vi "PID control XYZ R.vi"(0 "location":T2, 1 "x polarity":bool=TRUE, 2 "y polarity":bool, 3 "z polarity":bool, 5 "large deviation override":T1={"x (um)"=60.0, "y (um)"=80.0, "Poverride"=1.2}, 9 "deadband (um)":dbl=2.0, 11 "reinitialize? (F)":bool, 12 "XY pos range (um)":cluster{"output high":dbl, "output low":dbl}={"output high"=1000.0, "output low"=-1000.0} {"output low" format="%.2f"; "output high" format="%.2f"}, 13 "z position range (um)":cluster{"output high":dbl, "output low":dbl}={"output high"=100.0, "output low"=-100.0} {"output low" format="%.2f"; "output high" format="%.2f"}, 14 "XY gains":T3={"proportional gain (Kc)"=0.7, "integral time (Ti, sec)"=1.0, "derivative time (Td, sec)"=0.0} {"derivative time (Td, sec)" format="%.3f"; "integral time (Ti, sec)" format="%.3f"; "proportional gain (Kc)" format="%.3f"}, 15 "Z gains":T3={"proportional gain (Kc)"=0.7, "integral time (Ti, sec)"=1.0, "derivative time (Td, sec)"=0.0} {"derivative time (Td, sec)" format="%.3f"; "integral time (Ti, sec)" format="%.3f"; "proportional gain (Kc)" format="%.3f"}) -> (4 "x move (um)":dbl, 6 "y move (um)":dbl, 8 "z move (um)":dbl)   [LabVIEW 2010]
uses:
  location3D.ctl
  <vilib>/addons/control/pid/pid.llb/PID (DBL Array).vi
  <vilib>/addons/control/pid/NI_PID_pid.lvlib
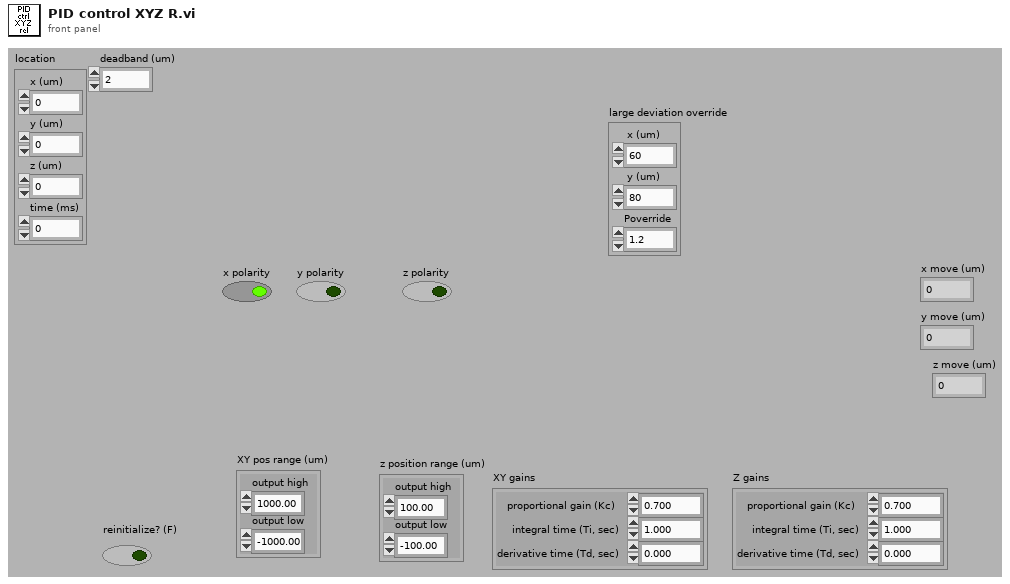
[diagram p1: front panel]
types:
  T1 = cluster{"x (um)":dbl, "y (um)":dbl, "Poverride":dbl}
  T2 = typedef "location3D.ctl" = cluster{"x (um)":dbl, "y (um)":dbl, "z (um)":dbl, "time (ms)":i64}
  T3 = cluster{"proportional gain (Kc)":dbl, "integral time (Ti, sec)":dbl, "derivative time (Td, sec)":dbl}
  T4 = cluster{"proportional gain (Kc)":dbl, "integral time (Ti, min)":dbl, "derivative time (Td, min)":dbl}
  T5 = cluster{"proportional gain (Kc)":dbl, "integral time (Ti, min)":dbl, "derivative time (Td, min)":dbl}[]
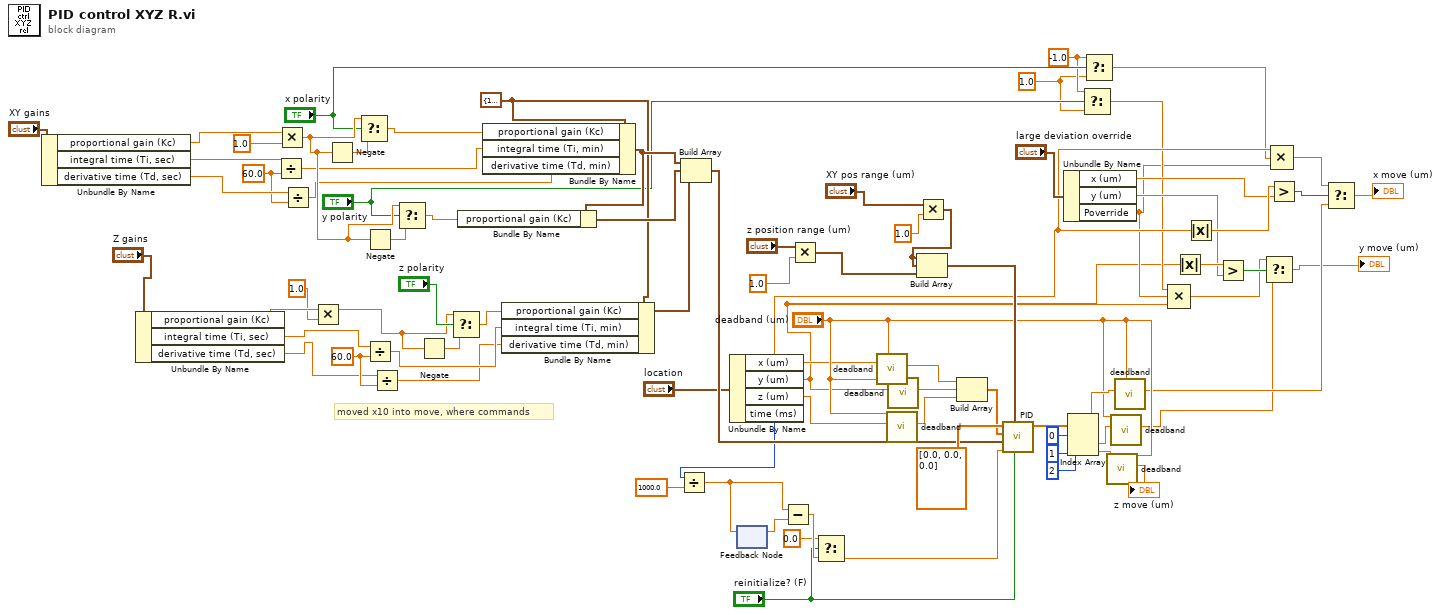
[diagram p0: block diagram]
diagram:
  w14 = 1.0 ("f")
  w15 = -1.0 ("t")
  w46 = 60.0 ("y")
  w77 = 60.0 ("y")
  w47 = T4 {"proportional gain (Kc)"=1.0, "integral time (Ti, min)"=0.01, "derivative time (Td, min)"=0.0} ("Z gains")
  # "moved x10 into move, where commands"
  n1 = Unbundle By Name("XY gains") -> ("proportional gain (Kc)"=w55:dbl, "integral time (Ti, sec)"=w79:dbl, "derivative time (Td, sec)"=w78:dbl)
  n2 = Unbundle By Name("Z gains") -> ("proportional gain (Kc)"=w51:dbl, "integral time (Ti, sec)"=w45:dbl, "derivative time (Td, sec)"=w44:dbl)
  n3 = Divide(x=w79, y=w77) -> (x/y=w72:dbl)
  n4 = Multiply(x=w55, y=1.0) -> (x*y=w74:dbl)
  n5 = Divide(x=w78, y=w77) -> (x/y=w71:dbl)
  n6 = Multiply(x=w51, y=1.0) -> (x*y=w49:dbl)
  n7 = Negate(x=w74) -> (-x=w76:dbl)
  n8 = Select(t=w74, s="x polarity", f=w76) -> (s? t:f=w73:dbl)
  n9 = Negate(x=w74) -> (-x=w75:dbl)
  n10 = Divide(x=w45, y=w46) -> (x/y=w43:dbl)
  n11 = Divide(x=w44, y=w46) -> (x/y=w42:dbl)
  n12 = Select(t=w74, s="y polarity", f=w75) -> (s? t:f=w70:dbl)
  n13 = Negate(x=w49) -> (-x=w52:dbl)
  n14 = Select(t=w49, s="z polarity", f=w52) -> (s? t:f=w50:dbl)
  n15 = Bundle By Name(cluster=w47, "proportional gain (Kc)"=w73, "integral time (Ti, min)"=w72, "derivative time (Td, min)"=w71) -> (w69:T4)
  n16 = Bundle By Name(cluster=w69, "proportional gain (Kc)"=w70) -> (w68:T4)
  n17 = Bundle By Name(cluster=w47, "proportional gain (Kc)"=w50, "integral time (Ti, min)"=w43, "derivative time (Td, min)"=w42) -> (w66:T4)
  n18 = Build Array(w69, w68, w66) -> (w65:T5)
  n19 = Unbundle By Name("location") -> ("x (um)"=w13:dbl, "y (um)"=w4:dbl, "z (um)"=w27:dbl, "time (ms)"=w26:i64)
  n20 = Divide(x=w26, y=1000.0) -> (x/y=w24:dbl)
  n21 = feedback-in #1(w24) -> ()
  n22 = feedback #1() -> (w82:dbl)  [unwired: 1 in]
  n23 = Subtract(x=w24, y=w82) -> (x-y=w81:dbl)
  n24 = Multiply(x="z position range (um)", y=1.0 ("measurement time")) -> (x*y=w62:cluster{"output high":dbl, "output low":dbl})
  n25 = Select(t=0.0, s="reinitialize? (F)", f=w81) -> (s? t:f=w38:dbl)
  n26 = call "deadband.vi"("minAbsX"="deadband (um)", "x"=w13) -> ("x out"=w35:dbl)  [unwired: 9 in]
  n27 = call "deadband.vi"("minAbsX"="deadband (um)", "x"=w27) -> ("x out"=w33:dbl)  [unwired: 9 in]
  n28 = call "deadband.vi"("minAbsX"="deadband (um)", "x"=w4) -> ("x out"=w34:dbl)  [unwired: 9 in]
  n29 = Multiply(x="XY pos range (um)", y=1.0 ("measurement time")) -> (x*y=w39:cluster{"output high":dbl, "output low":dbl})
  n30 = Build Array(w39, w39, w62) -> (w60:cluster{"output high":dbl, "output low":dbl}[])
  n31 = Build Array(w35, w34, w33) -> (w61:dbl[])
  n32 = call-poly <vilib>:"PID.vi"("reinitialize? (F)"="reinitialize? (F)", "output range"=w60, "dt (s)"=w38, "PID gains"=w65, "process variable"=w61, "setpoint"=dbl[] [0.0, 0.0, 0.0]) -> ("output"=w59:dbl[])  [unwired: 4 in, 1 out]
  n33 = Unbundle By Name("large deviation override") -> ("x (um)"=w19:dbl, "y (um)"=w18:dbl, "Poverride"=w5:dbl)
  n34 = Index Array(array=w59, index #1=0 ("index"), index #2=1 ("index"), index #3=2 ("index")) -> (element #1=w32:dbl, element #2=w31:dbl, element #3=w30:dbl)
  n35 = Select(t=w15, s="y polarity", f=w14) -> (s? t:f=w6:dbl)
  n36 = Select(t=w15, s="x polarity", f=w14) -> (s? t:f=w12:dbl)
  n37 = call "deadband.vi"("minAbsX"="deadband (um)", "x"=w30) -> ("x out"=→"z move (um)":dbl)  [unwired: 9 in]
  n38 = call "deadband.vi"("minAbsX"="deadband (um)", "x"=w31) -> ("x out"=w2:dbl)  [unwired: 9 in]
  n39 = call "deadband.vi"("minAbsX"="deadband (um)", "x"=w32) -> ("x out"=w9:dbl)  [unwired: 9 in]
  n40 = Compound Arithmetic op=MULTIPLY(w6, w5, w4) -> (w3:dbl)
  n41 = Absolute Value(x=w4) -> (abs(x)=w21:dbl)
  n42 = Absolute Value(x=w13) -> (abs(x)=w22:dbl)
  n43 = Greater?(x=w21, y=w18) -> (0:w7:bool)
  n44 = Select(t=w3, s=w7, f=w2) -> (s? t:f=→"y move (um)":dbl)
  n45 = Greater?(x=w22, y=w19) -> (0:w11:bool)
  n46 = Compound Arithmetic op=MULTIPLY(w13, w12, w5) -> (w10:dbl)
  n47 = Select(t=w10, s=w11, f=w9) -> (s? t:f=→"x move (um)":dbl)
